vi "LoadState.vi"   [LabVIEW 2016]
uses:
  TestControl.ctl
  SlobalState.vi
types:
  T1 = typedef "TestControl.ctl" = cluster{"Array":dbl[], "String":string, "Numeric":dbl, "Numeric 2":dbl}
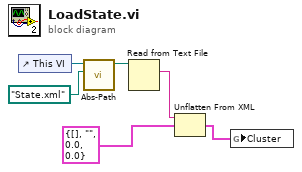
[diagram p0: block diagram]
diagram:
  n1 = control-ref of="This VI"() -> (w3:refnum<vi>)
  n2 = call "Abs-Path.vi"("filename"=path "State.xml" ("file (use dialog)"), "Vi in path"=w3) -> ("Full path"=w2:path)  [unwired: 9 in]
  n3 = Read from Text File(file (use dialog)=w2) -> (text=w6:string)  [unwired: 3 in, 3 out]
  n4 = Unflatten From XML(xml string=w6, type=T1 {"Array"=[], "String"="", "Numeric"=0.0, "Numeric 2"=0.0} ("Cluster")) -> (value=w1:T1)  [unwired: 1 in, 1 out]
  n5 = global write "SlobalState.vi" "Cluster"(w1) -> ()
